vi "Resolve Template Value.vi"(6 "Locals":map{string, string}(c390), 7 "Folder":path, 8 "error in (no error)":errorcluster, 9 "Template Service in":refnum<class "TemplateService.lvclass">, 10 "Value Name":string, 11 "TemplateVariableResolver in":refnum<class "TemplateValueResolver.lvclass">) -> (0 "error out":errorcluster, 1 "Template Service":refnum<class "TemplateService.lvclass">, 2 "Value":string)   [LabVIEW 2020, in "HTTP Server.lvlib" / "TemplateValueResolver.lvclass"]
uses:
  TemplateValueResolver.lvclass
  TemplateService/TemplateService.lvclass
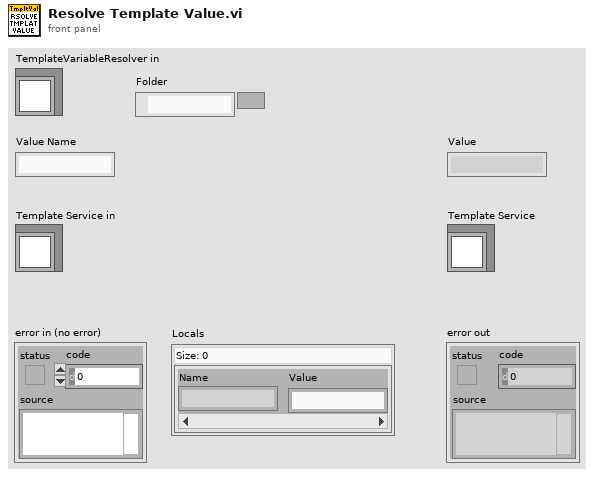
[diagram p1: front panel]
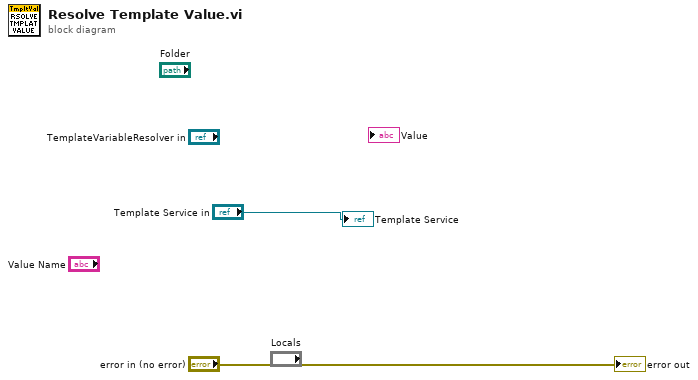
[diagram p0: block diagram]
diagram:
  "error out" <- "error in (no error)"
  "Template Service" <- "Template Service in"
